vi "Design IIR filter.vi"(4 "Optional IIR Filter Specifications":T4 {"PB Gain" format="%0.2f"; "SB Gain" format="%0.2f"; "Lower SB" format="%0.2p"; "Upper SB" format="%0.2f"; "Lower PB" format="%0.2p"; "Upper PB" format="%0.2f"}, 6 "IIR Filter specifications":T5 {"PB Ripple" format="%0.2f"; "Lower Fc" format="%0.2p"; "SB Attenuation" format="%0.2f"; "Upper Fc" format="%0.2p"}, 7 "Redesign filter":bool, 8 "error in":errorcluster, 10 "filter structure option":T1=10 items=["IIR 2nd Order"=0, "IIR 4th Order"=1, "Auto Select"=10], 11 "dt":dbl format="%0.2f") -> (0 "error out":errorcluster, 1 "IIR Filter Cluster":T2 {"Forward Coefficients" format="%0.2f"; "Reverse Coefficients" format="%0.2f"}, 3 "Filter Information":T3 {"phase H(w)"."df" format="%0.2f"; "phase H(w)"."f0" format="%0.2f"; "phase H(w)"."Phase H(w)" format="%0.2f"; "magnitude H(w)"."df" format="%0.2f"; "magnitude H(w)"."f0" format="%0.2f"; "magnitude H(w)"."Mag H(w)" format="%0.2f"}, 5 "Reset filter state":bool)   [LabVIEW 2020, in "NI_MAPro.lvlib"]
uses:
  NI_MAPro.lvlib
  Filter Structure Type.ctl
  NI_AALBase.lvlib
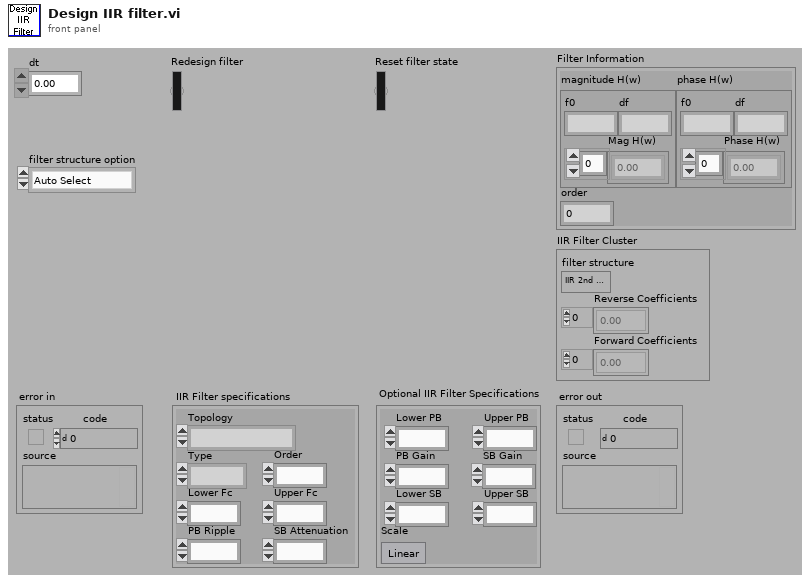
[diagram p1: front panel]
types:
  T1 = typedef "NI_AALBase.lvlib/Filter Structure Type.ctl" = u16
  T2 = cluster{"filter structure":enum32{"IIR 2nd Order", "IIR 4th Order"}, "Reverse Coefficients":dbl[], "Forward Coefficients":dbl[]}
  T3 = cluster{"magnitude H(w)":cluster{"f0":dbl, "df":dbl, "Mag H(w)":dbl[]}, "phase H(w)":cluster{"f0":dbl, "df":dbl, "Phase H(w)":dbl[]}, "order":i32}
  T4 = cluster{"Lower PB":dbl, "Upper PB":dbl, "Lower SB":dbl, "Upper SB":dbl, "PB Gain":dbl, "SB Gain":dbl, "Scale":bool}
  T5 = cluster{"Topology":enum16{"Off", "Butterworth", "Chebyshev", "Inverse Chebyshev", "Elliptic", "Bessel"}, "Type":enum16{"Lowpass", "Highpass", "Bandpass", "Bandstop"}, "Order":i32, "Lower Fc":dbl, "Upper Fc":dbl, "PB Ripple":dbl, "SB Attenuation":dbl}
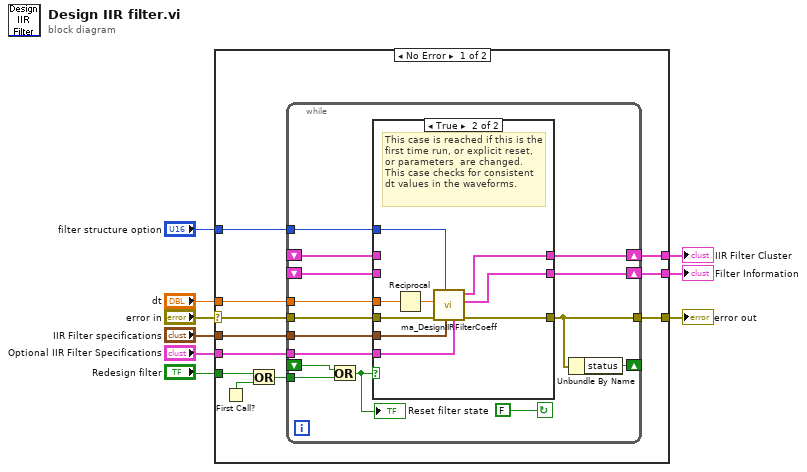
[diagram p0: block diagram]
diagram:
  n1 = case shown="No Error" "error in" {
    selector: "error in" -> [w19 w50]
    tunnel: [w20 w50] -> w9
    tunnel: [w18 T2 {"filter structure"=enum."IIR 2nd Order", "Reverse Coefficients"=[], "Forward Coefficients"=[]} ("IIR Filter Cluster")] -> w7
    tunnel: [w17 T3 {"magnitude H(w)"={"f0"=0.0, "df"=0.0, "Mag H(w)"=[]}, "phase H(w)"={"f0"=0.0, "df"=0.0, "Phase H(w)"=[]}, "order"=0} ("Filter Information")] -> w6
    tunnel: "filter structure option" -> [w14 _]
    tunnel: "dt" -> [w13 _]
    tunnel: "Redesign filter" -> [w12 _]
    tunnel: "Optional IIR Filter Specifications" -> [w11 _]
    tunnel: "IIR Filter specifications" -> [w10 _]
    frame No Error {
      n2 = First Call?() -> (First Call?: T/F=w16:bool)
      n3 = Or(x=w12, y=w16) -> (x .or. y?=w15:bool)
      n4 = while {
        tunnel: w11 -> [w28]
        tunnel: w10 -> [w29]
        tunnel: w13 -> [w30]
        tunnel: w19 -> [w27]
        tunnel: [w21] -> w20
        shift-left: _ -> [w32]
        shift-right: [w33] -> w17
        shift-left: _ -> [w35]
        shift-right: [w31] -> w18
        tunnel: w15 -> [w24]
        shift-right: [w26] -> _
        shift-left: _ -> [w25]
        tunnel: w14 -> [w22]
        stop <- FALSE continue-if-true
        n5 = Or(x=w25, y=w24) -> (x .or. y?=w23:bool)
        "Reset filter state" <- w23
        n6 = case shown="True" w23 {
          tunnel: w35 -> [w38 _]
          tunnel: [w37 w47] -> w33
          tunnel: w32 -> [w37 _]
          tunnel: [w38 w46] -> w31
          tunnel: [w36 w45] -> w21
          tunnel: w30 -> [_ w40]
          tunnel: w29 -> [_ w44]
          tunnel: w28 -> [_ w43]
          tunnel: w27 -> [w36 w42]
          tunnel: w22 -> [_ w39]
          frame False {
            # "No change in parameters, no reset, and not the first time run."
          }
          frame True {
            # "This case is reached if this is the first time run, or explicit reset, or parameters  are changed.  This case checks for consistent dt values in the waveforms."
            n7 = Reciprocal(x=w40) -> (1/x=w41:dbl)
            n8 = call "ma_DesignIIRFilterCoeff.vi"("Optional Filter Specifications"=w43, "Filter specifications"=w44, "filter structure option"=w39, "error in (no error)"=w42, "Sampling Frequency"=w41) -> ("error out"=w45:errorcluster, "Filter Information"=w47:T3, "IIR Filter Cluster"=w46:T2)  [unwired: 4 in]
          }
        }
        n9 = Unbundle By Name(w21) -> ("status"=w26:bool)
      }
    }
    frame Error {
    }
  }
  "error out" <- w9
  "IIR Filter Cluster" <- w7
  "Filter Information" <- w6
